vi "dvp Vi Get Frames Per Trigger.vi"(10 "pFramesPerTrigger":i32, 11 "handle":u32) -> (2 "pFramesPerTrigger out":i32, 3 "function return":u32(ring))   [LabVIEW 2018, in "LabViewDVPCamera.lvlib"]
doc: "LabviewDvp2Api dvpStatus dvpViGetFramesPerTrigger(dvpHandle handle, dvpInt32 *pFramesPerTrigger);"
uses:
  LabViewDVPCamera.lvlib
  LabViewDVPCamera/LabViewDVPCamera.dll
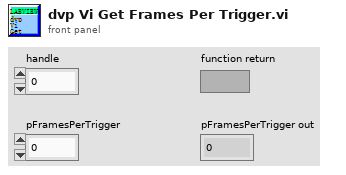
[diagram p1: front panel]
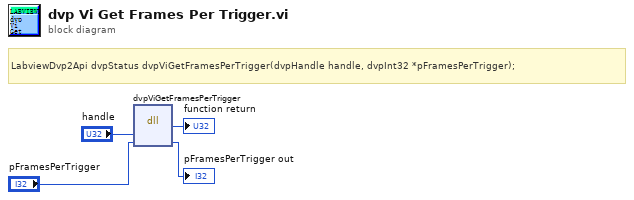
[diagram p0: block diagram]
diagram:
  # "LabviewDvp2Api dvpStatus dvpViGetFramesPerTrigger(dvpHandle handle, dvpInt32 *pFramesPerTrigger);"
  n1 = dll-call lib="C:/Program Files (x86)/DVP2 Labview cn 64/Sample/LabViewDVPCamera/LabViewDVPCamera.*" fn="dvpViGetFramesPerTrigger"("handle"="handle", "pFramesPerTrigger"="pFramesPerTrigger") -> (→"function return":u32, "pFramesPerTrigger"=→"pFramesPerTrigger out":i32)  [unwired: 4 in, 2 out]
